vi "ReadValue_Control1.vi"(11 "reference":refnum<vi>) -> (2 "value":T1)   [LabVIEW 2012]
uses:
  Typedefs/Control 1.ctl
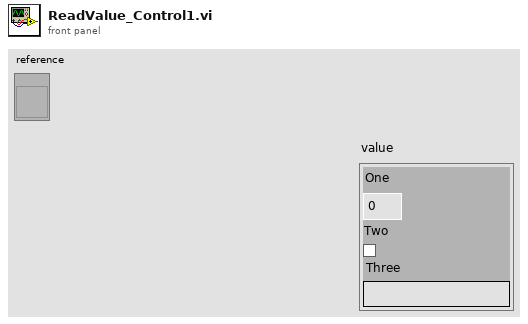
[diagram p1: front panel]
types:
  T1 = typedef "Control 1.ctl" = cluster{"One":dbl, "Two":bool, "Three":string}
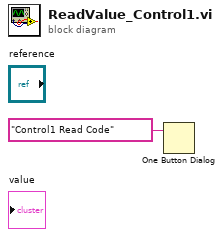
[diagram p0: block diagram]
diagram:
  n1 = One Button Dialog(message="Control1 Read Code" ("button name (\"OK\")")) -> ()  [unwired: 1 in, 1 out]
